vi "Parse NT Boolean Array.vi"(11 "TCP Network Connection in":refnum<k5>) -> (0 "String":string, 1 "Size":i32=1, 2 "Boolean Array":bool[](array[boolean]), 3 "TCP Network Connection out":refnum<k5>)   [LabVIEW 2017]
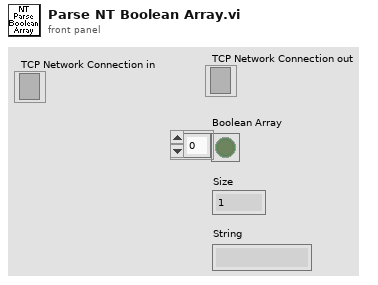
[diagram p1: front panel]
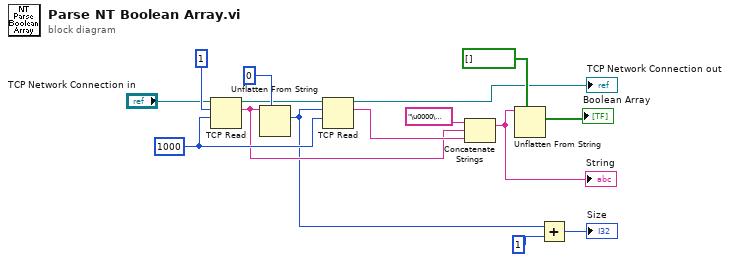
[diagram p0: block diagram]
diagram:
  w7 = 1000 ("timeout ms (25000)")
  n1 = TCP Read(connection ID="TCP Network Connection in", bytes to read=1 ("timeout ms (25000)"), 9:w7) -> (connection ID out=w9:refnum<k5>, data out=w5:string)  [unwired: 2 in, 1 out]
  n2 = Unflatten From String(type=u8 0 ("Size"), binary string=w5) -> (value=w1:u8)  [unwired: 3 in, 2 out]
  n3 = TCP Read(connection ID=w9, bytes to read=w1, 9:w7) -> (connection ID out=→"TCP Network Connection out":refnum<k5>, data out=w6:string)  [unwired: 2 in, 1 out]
  n4 = Concatenate Strings("\u0000\u0000\u0000", w5, w6) -> (w4:string)
  "String" <- w4
  n5 = Unflatten From String(type=bool[] [], binary string=w4) -> (value=→"Boolean Array":bool[])  [unwired: 3 in, 2 out]
  n6 = Add(x=w1, y=u8 1 ("timeout ms (25000)")) -> (x+y=→"Size":u8)
